vi "Pockels Cal-Set graph cursors.vi"(5 "Function":T2(ring), 7 "Cal subset indexes":T1={"Start point index"=0, "End point index"=11}, 8 "error in (no error)":errorcluster, 9 "Waveforms array":cluster{cluster{"X":dbl, "Y":dbl}[]}[](array[cluster])=[{[{"X"=0.0, "Y"=0.0}, {"X"=1.0, "Y"=10.0}, {"X"=2.0, "Y"=30.0}, {"X"=3.0, "Y"=50.0}, {"X"=4.0, "Y"=70.0}, {"X"=5.0, "Y"=90.0}, {"X"=6.0, "Y"=110.0}, {"X"=7.0, "Y"=130.0}, {"X"=8.0, "Y"=150.0}, {"X"=9.0, "Y"=181.0}, {"X"=10.0, "Y"=191.0}, {"X"=11.0, "Y"=195.0}, {"X"=12.0, "Y"=230.0}, {"X"=13.0, "Y"=250.0}, {"X"=14.0, "Y"=270.0}, {"X"=15.0, "Y"=300.0}]}], 11 "XYGraph in":refnum<vi>) -> (0 "error out":errorcluster, 3 "XYGraph out":refnum<vi>)   [LabVIEW 2020]
panel:
  out "Number of equals":i32
  out "Index of plateau start":i32
  out "End point index":i32
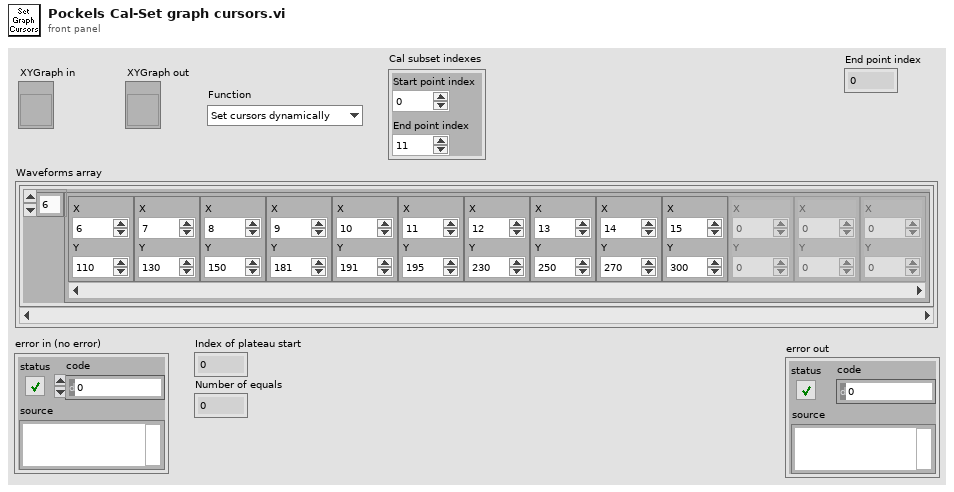
[diagram p1: front panel]
types:
  T1 = cluster{"Start point index":i32, "End point index":i32}
  T2 = enum16{"Set cursors dynamically", "Set cursors from file"}
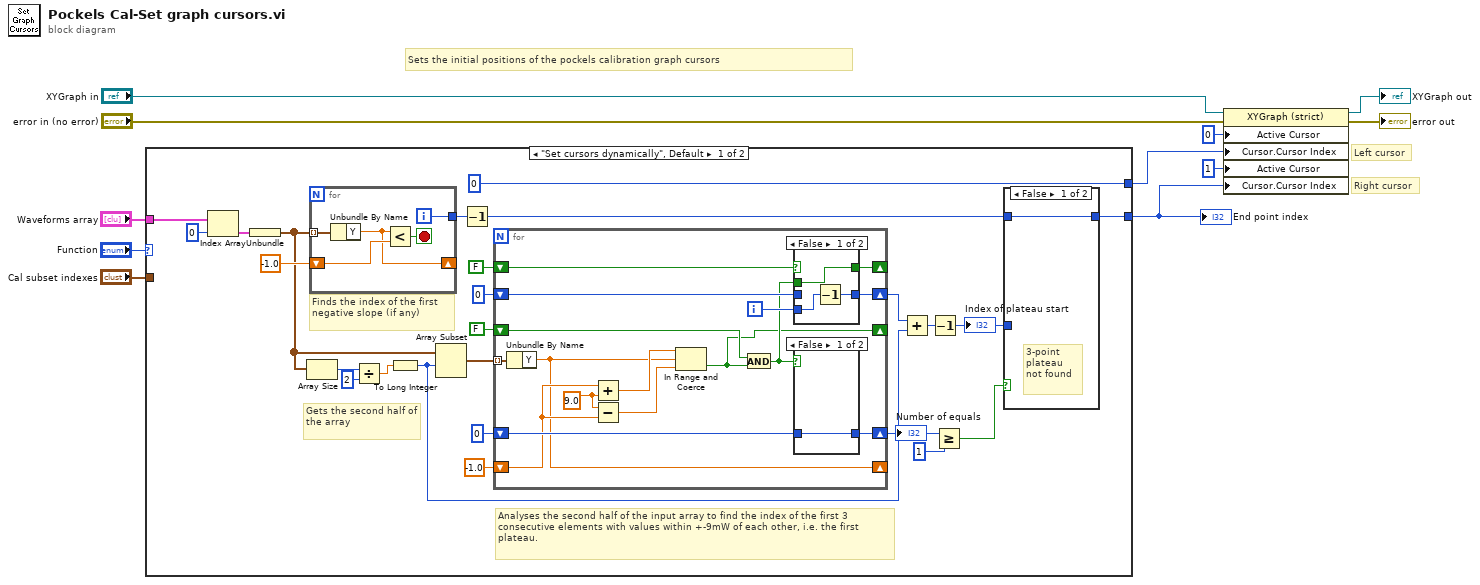
[diagram p0: block diagram]
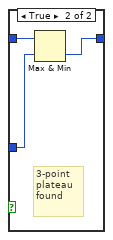
[diagram p2: hidden frame]
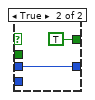
[diagram p3: hidden frame]
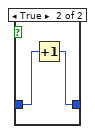
[diagram p4: hidden frame]
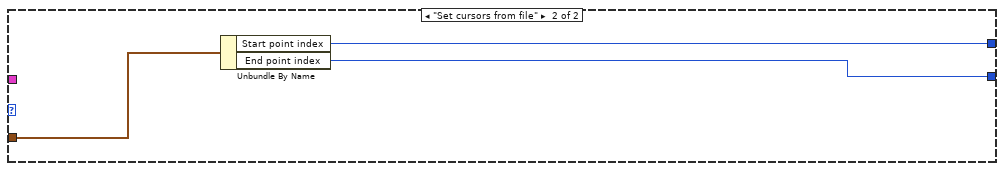
[diagram p5: hidden frame]
diagram:
  # "Left cursor"
  # "Right cursor"
  # "Sets the initial positions of the pockels calibration graph cursors"
  n1 = case shown="\"Set cursors dynamically\", Default" "Function" {
    tunnel: [0 ("Cursor.Cursor Index") w71] -> w11
    tunnel: "Waveforms array" -> [w34 _]
    tunnel: [w14 w70] -> w3
    tunnel: "Cal subset indexes" -> [_ w72]
    frame "Set cursors dynamically", Default {
      # "Analyses the second half of the input array to find the index of the first 3 consecutive elements with values within +-9mW of each other, i.e. the first plateau."
      # "Gets the second half of the array"
      # "Finds the index of the first negative slope (if any)"
      n2 = Index Array(array=w34, index=0) -> (element=w35:cluster{cluster{"X":dbl, "Y":dbl}[]})
      n3 = Unbundle(w35) -> (w28:cluster{"X":dbl, "Y":dbl}[])
      n4 = Array Size(array=w28) -> (size(s)=w30:i32)
      n5 = for {
        tunnel: w28 -> [w69] mode=indexing
        tunnel: [w66] -> w32
        shift-right: [w65] -> _
        shift-left: -1.0 ("y") -> [w68]
        i -> [w66]
        stop <- w67 stop-if-true
        n6 = Unbundle By Name(w69) -> ("Y"=w65:dbl)
        n7 = Less?(x=w65, y=w68) -> (x < y?=w67:bool)
      }
      n8 = Divide(x=w30, y=2) -> (x/y=w27:dbl)
      n9 = To Long Integer(number=w27) -> (32bit integer=w23:i32)
      n10 = Array Subset(array=w28, index=w23) -> (w26:cluster{"X":dbl, "Y":dbl}[])  [unwired: 1 in]
      n11 = Decrement(x=w32) -> (x-1=w15:i32)
      n12 = for {
        tunnel: w26 -> [w56] mode=indexing
        shift-right: [w41] -> _
        shift-left: -1.0 ("Y") -> [w44]
        shift-right: [w54] -> w18
        shift-left: 0 ("Cursor.Cursor Index") -> [w55]
        shift-right: [w52] -> w19
        shift-left: 0 -> [w50]
        shift-right: [w49] -> _
        shift-left: FALSE -> [w53]
        shift-right: [w46] -> _
        shift-left: FALSE -> [w47]
        i -> [w51]
        w45 = 9.0
        n13 = Unbundle By Name(w56) -> ("Y"=w41:dbl)
        n14 = Add(x=w44, y=w45) -> (x+y=w43:dbl)
        n15 = Subtract(x=w45, y=w44) -> (x-y=w42:dbl)
        n16 = In Range and Coerce(upper limit=w43, x=w41, lower limit=w42) -> (In Range?=w46:bool)  [unwired: 1 out]
        n17 = And(x=w47, y=w46) -> (x .and. y?=w48:bool)
        n18 = case shown="False" w53 {
          tunnel: [w57 w61] -> w52
          tunnel: w51 -> [w58 _]
          tunnel: w50 -> [_ w61]
          tunnel: [w59 TRUE] -> w49
          tunnel: w48 -> [w59 _]
          frame False {
            n19 = Decrement(x=w58) -> (x-1=w57:i32)
          }
          frame True {
          }
        }
        n20 = case shown="False" w48 {
          tunnel: w55 -> [w62 w64]
          tunnel: [w62 w63] -> w54
          frame False {
          }
          frame True {
            n21 = Increment(x=w64) -> (x+1=w63:i32)
          }
        }
      }
      "Number of equals" <- w18
      n22 = Add(x=w19, y=w23) -> (x+y=w22:i32)
      n23 = Decrement(x=w22) -> (x-1=w13:i32)
      "Index of plateau start" <- w13
      n24 = Greater Or Equal?(x=w18, y=1) -> (x >= y?=w16:bool)
      n25 = case shown="False" w16 {
        tunnel: w15 -> [w37 w40]
        tunnel: [w37 w38] -> w14
        tunnel: w13 -> [_ w39]
        frame False {
          # "3-point plateau not found"
        }
        frame True {
          # "3-point plateau found"
          n26 = Max & Min(x=w40, y=w39) -> (min(x,y)=w38:i32)  [unwired: 1 out]
        }
      }
    }
    frame "Set cursors from file" {
      n27 = Unbundle By Name(w72) -> ("Start point index"=w71:i32, "End point index"=w70:i32)
    }
  }
  "End point index" <- w3
  n28 = property on="Property Node" class="XYGraph (strict)"(reference="XYGraph in", error in="error in (no error)", "Active Cursor"=u32 0, "Cursor.Cursor Index"=w11, "Active Cursor"=u32 1, "Cursor.Cursor Index"=w3) -> (reference out=→"XYGraph out":refnum<vi>, error out=→"error out":errorcluster)
